vi "Read assemblies.vi"(8 "error in":errorcluster, 11 "EthernetIP configuration in":refnum<class "EthernetIP configuration.lvclass">) -> (0 "error out":errorcluster, 2 "assemblies":T1[](array[typedef]), 3 "EthernetIP configuration out":refnum<class "EthernetIP configuration.lvclass">)   [LabVIEW 2013, in "EthernetIP configuration.lvclass"]
uses:
  EthernetIP configuration.lvclass
  assembly definition.ctl
  assembly type.ctl
  EthernetIP configuration.lvclass/EthernetIP configuration.ctl
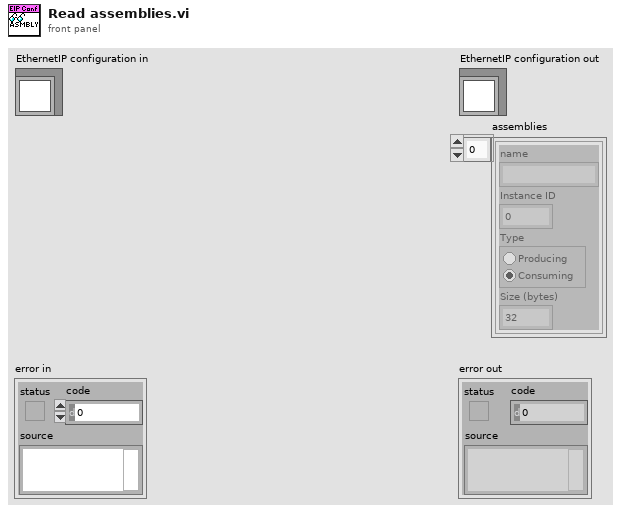
[diagram p1: front panel]
types:
  T1 = typedef "EthernetIP configuration.lvclass/assembly definition.ctl" = cluster{"name":string, "Instance ID":u32, "Type":T2, "Size (bytes)":u32}
  T2 = typedef "EthernetIP configuration.lvclass/assembly type.ctl" = enum32{"Producing", "Consuming"}
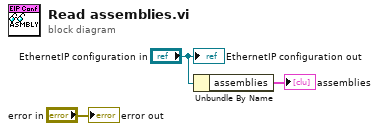
[diagram p0: block diagram]
diagram:
  n1 = Unbundle By Name("EthernetIP configuration in") -> ("assemblies"=→"assemblies":T1[])
  "error out" <- "error in"
  "EthernetIP configuration out" <- "EthernetIP configuration in"
